vi "solar_misc Email Dialog.vi"(8 "error in (no error)":errorcluster, 11 "EmailConfig in":T1={"Enabled"=FALSE, "MailServer"="mail.aero.ball.com", "MailServerPort"=25, "EmailTimeout"=5000, "ReturnAddress"="batcsolar@ball.com", "Recipients"=[], "Subject"=""}) -> (0 "error out":errorcluster, 1 "Cancelled?":bool, 3 "EmailConfig out":T1={"Enabled"=FALSE, "MailServer"="mail.aero.ball.com", "MailServerPort"=25, "EmailTimeout"=5000, "ReturnAddress"="batcsolar@ball.com", "Recipients"=[], "Subject"=""})   [LabVIEW 2018]
doc: "This VI is a dialog to configure the Email settings."
uses:
  solar_misc_ctl Email Config.ctl
panel:
  in  "TestEmail":bool
  out "TestSent":string
  in  "Subject":string
  in  "Recipients":string[](array[string])
  in  "Enabled":enum32{"Disabled", "Enabled"}(radio) caption="Notifications"
  in  "EmailTimeout":i32=5000 caption="TCP Timeout" format="%d ms"
  in  "ReturnAddress":string="batcsolar@ball.com" caption="Return Address"
  in  "MailServerPort":u16=25 caption="Port"
  in  "MailServer":string="mail.aero.ball.com" caption="Mail Server"
  in  "Cancel":bool
  in  "OK":bool
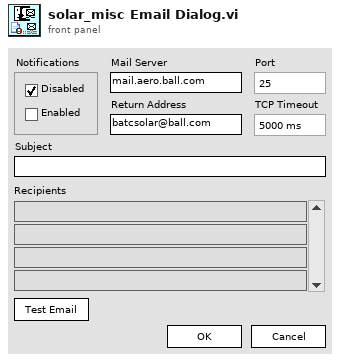
[diagram p1: front panel]
types:
  T1 = typedef "solar_misc_ctl Email Config.ctl" = cluster{"Enabled":bool, "MailServer":string, "MailServerPort":u16, "EmailTimeout":i32, "ReturnAddress":string, "Recipients":string[], "Subject":string}
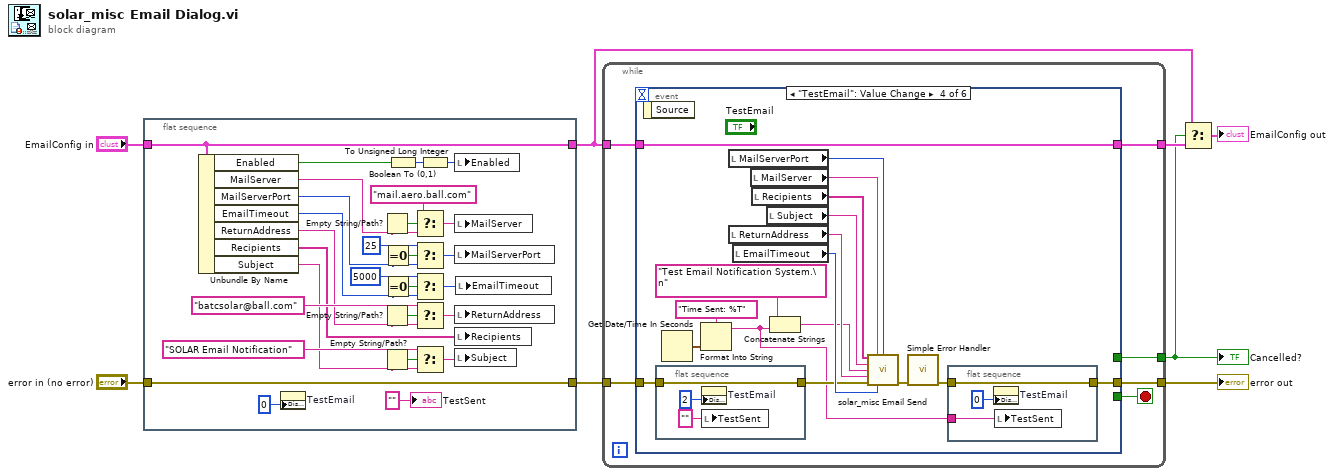
[diagram p0: block diagram]
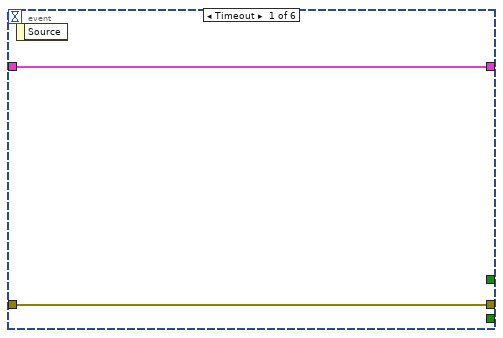
[diagram p2: hidden frame]
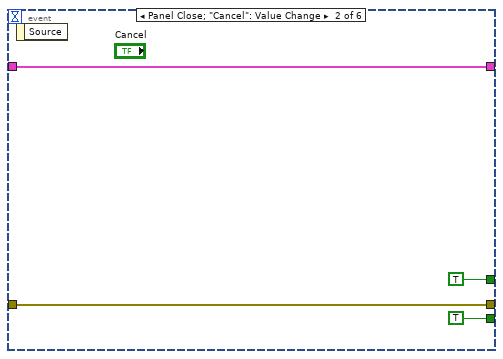
[diagram p3: hidden frame]
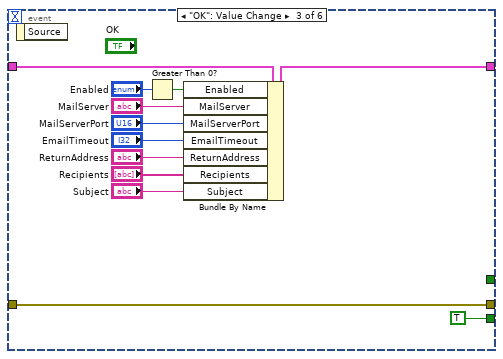
[diagram p4: hidden frame]
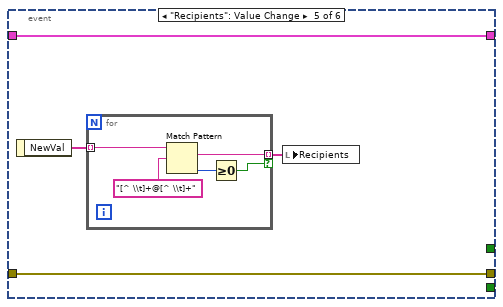
[diagram p5: hidden frame]
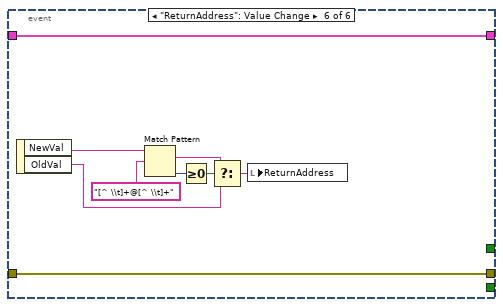
[diagram p6: hidden frame]
diagram:
  n1 = flat-sequence {
    tunnel: "error in (no error)" -> [w19]
    tunnel: [w19] -> w6
    tunnel: "EmailConfig in" -> [w11]
    tunnel: [w11] -> w2
    frame #0 {
      n2 = Unbundle By Name(w11) -> ("Enabled"=w18:bool, "MailServer"=w17:string, "MailServerPort"=w16:u16, "EmailTimeout"=w15:i32, "ReturnAddress"=w14:string, "Recipients"=w13:string[], "Subject"=w12:string)
      n3 = property on="TestEmail" class="Bool"("DisabledEnum"=u8 0) -> ()  [unwired: 2 in, 2 out]
      n4 = Empty String/Path?(string/path=w17) -> (empty?=w34:bool)
      n5 = Empty String/Path?(string/path=w14) -> (empty?=w25:bool)
      n6 = Empty String/Path?(string/path=w12) -> (empty?=w22:bool)
      n7 = Equal To 0?(x=w16) -> (x = 0?=w31:bool)
      n8 = Equal To 0?(x=w15) -> (x = 0?=w27:bool)
      n9 = Boolean To (0,1)(Boolean=w18) -> (0, 1=w36:i16)
      n10 = Select(t="mail.aero.ball.com", s=w34, f=w17) -> (s? t:f=w32:string)
      n11 = Select(t=u16 25, s=w31, f=w16) -> (s? t:f=w29:u16)
      n12 = Select(t=5000, s=w27, f=w15) -> (s? t:f=w26:i32)
      n13 = Select(t="batcsolar@ball.com", s=w25, f=w14) -> (s? t:f=w24:string)
      n14 = Select(t="SOLAR Email Notification", s=w22, f=w12) -> (s? t:f=w21:string)
      n15 = To Unsigned Long Integer(number=w36) -> (unsigned 32bit integer=w35:u32)
      n16 = local write "Enabled"(w35) -> ()
      n17 = local write "MailServer"(w32) -> ()
      n18 = local write "MailServerPort"(w29) -> ()
      n19 = local write "ReturnAddress"(w24) -> ()
      n20 = local write "Recipients"(w13) -> ()
      n21 = local write "Subject"(w21) -> ()
      n22 = local write "EmailTimeout"(w26) -> ()
      "TestSent" <- "" ("TestSent")
    }
  }
  n23 = while {
    tunnel: [w41] -> w8
    tunnel: w6 -> [w40]
    tunnel: [w39] -> w3
    tunnel: w2 -> [w38]
    tunnel: [w37] -> w4
    stop <- w42 stop-if-true
    n24 = event shown="[3] \"TestEmail\": Value Change" {
      selector: _ -> [_ _ _ _ _ _]
      dyn-events: _ -> [_ _ _ _ _ _]
      timeout: _ -> [_ _ _ _ _ _]
      tunnel: [_ TRUE TRUE _ _ _] -> w42
      tunnel: [w44 w47 w51 w64 w87 w101] -> w41
      tunnel: w40 -> [w44 w47 w51 w66 w87 w101]
      tunnel: [_ TRUE _ _ _ _] -> w39
      tunnel: w38 -> [w43 w45 w50 w68 w84 w93]
      tunnel: [w43 w45 w49 w68 w84 w93] -> w37
      event Timeout {
        n25 = event-data() -> ()  [unwired: 1 in, 1 out]
      }
      event Panel Close; "Cancel": Value Change {
        n26 = event-data() -> ()  [unwired: 1 in, 1 out]
      }
      event "OK": Value Change {
        n27 = event-data() -> ()  [unwired: 1 in, 1 out]
        n28 = Greater Than 0?(x="Enabled") -> (x > 0?=w52:bool)
        n29 = Bundle By Name(cluster=w50, "Enabled"=w52, "MailServer"="MailServer", "MailServerPort"="MailServerPort", "EmailTimeout"="EmailTimeout", "ReturnAddress"="ReturnAddress", "Recipients"="Recipients", "Subject"="Subject") -> (w49:T1)
      }
      event "TestEmail": Value Change {
        n30 = event-data() -> ()  [unwired: 1 in, 1 out]
        n31 = flat-sequence {
          tunnel: [w82] -> w67
          tunnel: w66 -> [w82]
          frame #0 {
            n32 = property on="TestEmail" class="Bool"("DisabledEnum"=u8 2) -> ()  [unwired: 2 in, 2 out]
            n33 = local write "TestSent"("" ("TestSent")) -> ()
          }
        }
        n34 = Get Date/Time In Seconds() -> (seconds since 1Jan1904=w75:timestamp)
        n35 = Format Into String(format string="Time Sent: %T" ("Subject"), w75) -> (resulting string=w61:string)  [unwired: 2 in, 1 out]
        n36 = local read "MailServerPort"() -> (w71:u16)
        n37 = local read "ReturnAddress"() -> (w74:string)
        n38 = local read "EmailTimeout"() -> (w73:i32)
        n39 = local read "MailServer"() -> (w72:string)
        n40 = local read "Recipients"() -> (w77:string[])
        n41 = local read "Subject"() -> (w70:string)
        n42 = Concatenate Strings("Test Email Notification System.\n" ("Subject"), w61) -> (w62:string)
        n43 = call "solar_misc Email Send.vi"("Recipients"=w77, "Mail Server (\"mail.aero.ball.com\")"=w72, "Mail Server Port (25)"=w71, "Subject"=w70, "Message"=w62, "Return Address"=w74, "error in (no error)"=w67, "TCP Timeout (5000ms)"=w73) -> ("error out"=w69:errorcluster)  [unwired: 5 in, 2 out]
        n44 = call <vilib>:"Simple Error Handler.vi"("error in (no error)"=w69) -> ("error out"=w65:errorcluster)  [unwired: 4 in, 4 out]
        n45 = flat-sequence {
          tunnel: [w79] -> w64
          tunnel: w65 -> [w79]
          tunnel: w61 -> [w78]
          frame #0 {
            n46 = property on="TestEmail" class="Bool"("DisabledEnum"=u8 0) -> ()  [unwired: 2 in, 2 out]
            n47 = local write "TestSent"(w78) -> ()
          }
        }
      }
      event "Recipients": Value Change {
        n48 = event-data() -> ("NewVal"=w86:string[])  [unwired: 1 in]
        n49 = for {
          tunnel: w86 -> [w92] mode=indexing
          tunnel: [w89] -> w85 mode=indexing if=w88
          n50 = Match Pattern(string=w92, regular expression="[^ \\t]+@[^ \\t]+") -> (match substring=w89:string, offset past match=w90:i32)  [unwired: 1 in, 2 out]
          n51 = Greater Or Equal To 0?(x=w90) -> (x >= 0?=w88:bool)
        }
        n52 = local write "Recipients"(w85) -> ()
      }
      event "ReturnAddress": Value Change {
        n53 = event-data() -> ("NewVal"=w97:string, "OldVal"=w95:string)  [unwired: 1 in]
        n54 = Match Pattern(string=w97, regular expression="[^ \\t]+@[^ \\t]+") -> (match substring=w96:string, offset past match=w99:i32)  [unwired: 1 in, 2 out]
        n55 = Greater Or Equal To 0?(x=w99) -> (x >= 0?=w98:bool)
        n56 = Select(t=w96, s=w98, f=w95) -> (s? t:f=w94:string)
        n57 = local write "ReturnAddress"(w94) -> ()
      }
    }
  }
  "error out" <- w8
  "Cancelled?" <- w3
  n58 = Select(t=w2, s=w3, f=w4) -> (s? t:f=→"EmailConfig out":T1)
